vi "UpdateTriggerControl.vi"(8 "error in (no error)":errorcluster, 9 "Device":string, 10 "Varialbe":string="Trigger.Mode", 11 "RingRef":refnum<vi>) -> (0 "error IO":errorcluster)   [LabVIEW 2013]
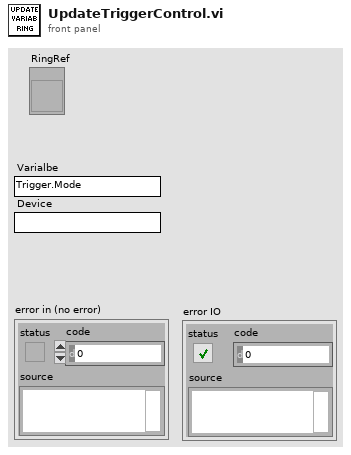
[diagram p1: front panel]
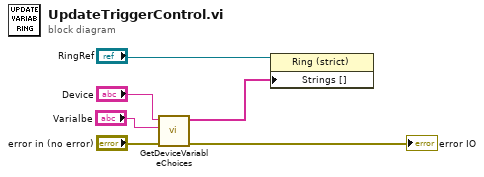
[diagram p0: block diagram]
diagram:
  n1 = call "GetDeviceVariableChoices.vi"("error in (no error)"="error in (no error)", "element"="Varialbe", "Device/Devicetype name\n/Plotter.id/ScanName#"="Device") -> ("error IO"=→"error IO":errorcluster, "Choiches[]"=w3:string[])  [unwired: 7 in]
  n2 = property class="Ring (strict)"(reference="RingRef", "Strings []"=w3) -> ()  [unwired: 1 in, 2 out]
